vi "Buffered String FGV.vi"(6 "Reset":bool, 11 "String":string) -> ()   [LabVIEW 2017]
panel:
  out "Strings":string
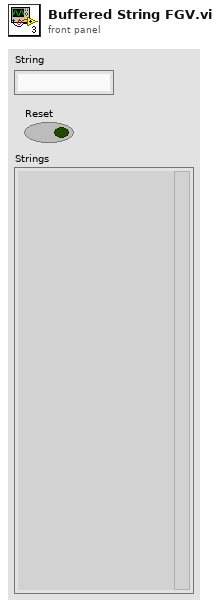
[diagram p1: front panel]
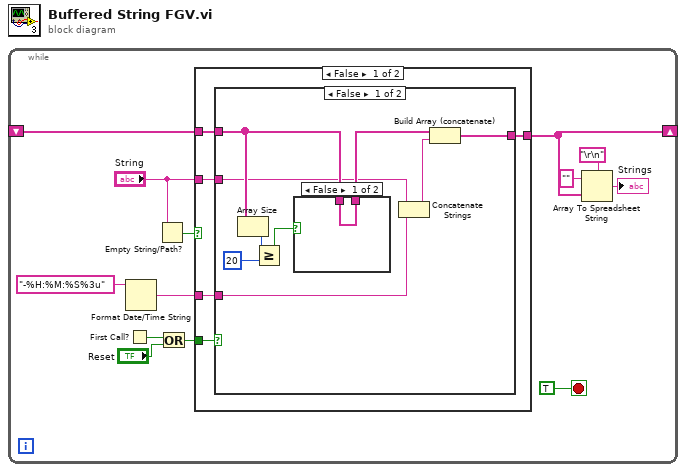
[diagram p0: block diagram]
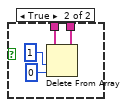
[diagram p2: hidden frame]
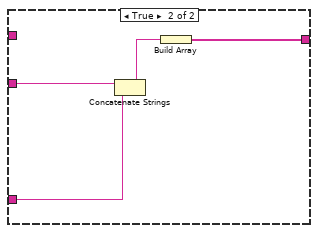
[diagram p3: hidden frame]
diagram:
  n1 = while {
    shift-right: [w8] -> _
    shift-left: _ -> [w9]
    stop <- TRUE stop-if-true
    n2 = First Call?() -> (First Call?: T/F=w11:bool)
    n3 = Format Date/Time String(time format string (%c)="-%H:%M:%S%3u") -> (date/time string=w1:string)  [unwired: 2 in]
    n4 = Empty String/Path?(string/path="String") -> (empty?=w4:bool)
    n5 = Or(x=w11, y="Reset") -> (x .or. y?=w12:bool)
    n6 = case shown="False" w4 {
      tunnel: w12 -> [w18 _]
      tunnel: w9 -> [w17 w37]
      tunnel: "String" -> [w16 _]
      tunnel: [w15 w37] -> w8
      tunnel: w1 -> [w14 _]
      frame False {
        n7 = case shown="False" w18 {
          tunnel: w17 -> [w26 _]
          tunnel: w16 -> [w21 w35]
          tunnel: [w27 w36] -> w15
          tunnel: w14 -> [w20 w33]
          frame False {
            n8 = Array Size(array=w26) -> (size(s)=w24:i32)
            n9 = Greater Or Equal?(x=w24, y=20) -> (x >= y?=w22:bool)
            n10 = case shown="False" w22 {
              tunnel: w26 -> [w28 w32]
              tunnel: [w28 w31] -> w25
              frame False {
              }
              frame True {
                n11 = Delete From Array(array=w32, length=1, index=0) -> (array with subset deleted=w31:string[])  [unwired: 1 out]
              }
            }
            n12 = Concatenate Strings(w21, w20) -> (w19:string)
            n13 = Build Array (concatenate)(w25, w19) -> (w27:string[])
          }
          frame True {
            n14 = Concatenate Strings(w35, w33) -> (w34:string)
            n15 = Build Array(w34) -> (w36:string[])
          }
        }
      }
      frame True {
      }
    }
    n16 = Array To Spreadsheet String(delimiter (Tab)="\r\n", array=w8, 3:"" ("format string")) -> (spreadsheet string=→"Strings":string)
  }
